vi "_Write.vi"(8 "error in (no error)":errorcluster, 9 "Timeout S (0)":dbl, 10 "Data":string, 11 "DeployResource in":refnum<class "Resource.lvclass">) -> (0 "error out":errorcluster, 2 "Bytes Written":i32, 3 "DeployResource out":refnum<class "Resource.lvclass">)   [LabVIEW 2020]
uses:
  Resource.lvclass/Resource.ctl
  Resource.lvclass
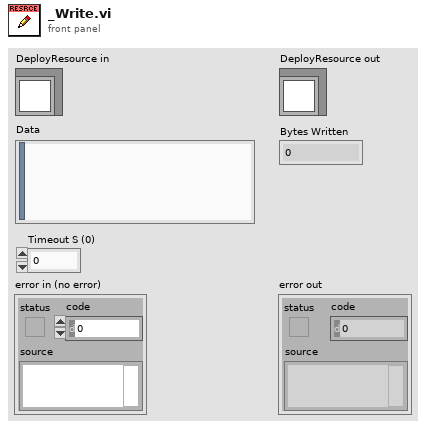
[diagram p1: front panel]
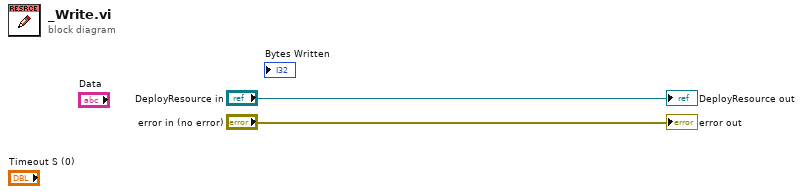
[diagram p0: block diagram]
diagram:
  "error out" <- "error in (no error)"
  "DeployResource out" <- "DeployResource in"
